vi "Read Failed Count.vi"(11 "Test Case Result In":T1) -> (2 "Fail count":i32, 3 "Test Case Result Out":T1)   [LabVIEW 2020, in "Test Case Result.lvlib"]
uses:
  Test Case Result.lvlib
  Test Case Result.ctl
  Method Result/Method Result.ctl
  Assertion Result/Public/TypeDefs/Status.ctl
  Assertion Result/Assertion Result.ctl
  Assertion Result/Public/TypeDefs/Assertion Type.ctl
  Assertion Result/Assertion Result.lvlib
  Method Result/Method Result.lvlib
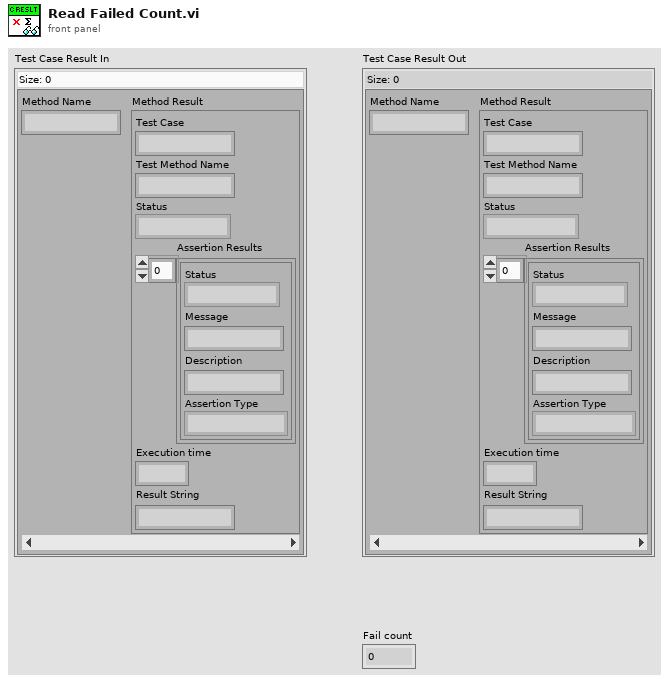
[diagram p1: front panel]
types:
  T1 = typedef "Test Case Result.lvlib/Test Case Result.ctl" = map{string, T2}
  T2 = typedef "Method Result.lvlib/Method Result.ctl" = cluster{"Test Case":string, "Test Method Name":string, "Status":T3, "Assertion Results":T4[], "Execution time":dbl, "Result String":string}
  T3 = typedef "Assertion Result.lvlib/Status.ctl" = enum16{"Pass", "Fail", "Error", "Skipped", "Setup Error", "Broken", "Teardown Error"}
  T4 = typedef "Assertion Result.lvlib/Assertion Result.ctl" = cluster{"Status":T3, "Message":string, "Description":string, "Assertion Type":T5}
  T5 = typedef "Assertion Result.lvlib/Assertion Type.ctl" = enum16{"None", "Pass", "Fail", "Skip", "Pass if Equal", "Fail if Equal", "Pass if Error", "Fail if Error", "Pass if", "Fail if"}
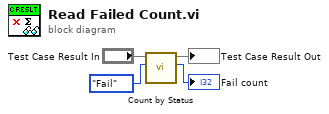
[diagram p0: block diagram]
diagram:
  n1 = call "Count by Status.vi"("Status"=Status."Fail", "Test Case Result In"="Test Case Result In") -> ("Count"=→"Fail count":i32, "Test Case Result Out"=→"Test Case Result Out":T1)  [unwired: 8 in]
